vi "From JSON.vi"(8 "error in (no error)":errorcluster, 10 "JSON":string, 11 "Type in":refnum<class "Abs_Value.lvclass">) -> (0 "error out":errorcluster, 3 "Type out":refnum<class "Abs_Value.lvclass">)   [LabVIEW 2021, in "Abs_Value.lvclass"]
uses:
  Abs_Value.lvclass
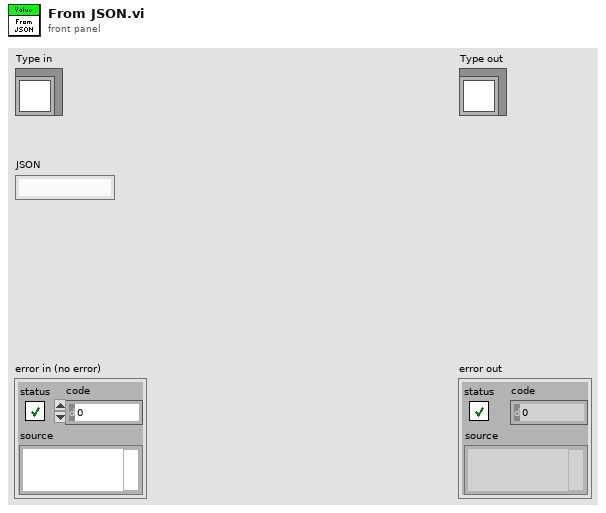
[diagram p1: front panel]
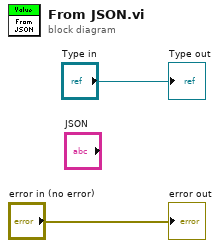
[diagram p0: block diagram]
diagram:
  "error out" <- "error in (no error)"
  "Type out" <- "Type in"
